vi "PWM Set Phase.vi"(8 "error in (no error)":errorcluster, 9 "pPhase":u16, 10 "ChannelMask":u8, 11 "DevHandle":i32) -> (0 "error out":errorcluster, 1 "pPhase out":u16, 3 "function return":i32)   [LabVIEW 2010, in "usb2pwm.lvlib"]
doc: "int WINAPI PWM_SetPhase(int DevHandle,unsigned char ChannelMask,unsigned short *pPhase);"
uses:
  usb2pwm.lvlib
  libs/msvc_x86/USB2XXX.dll
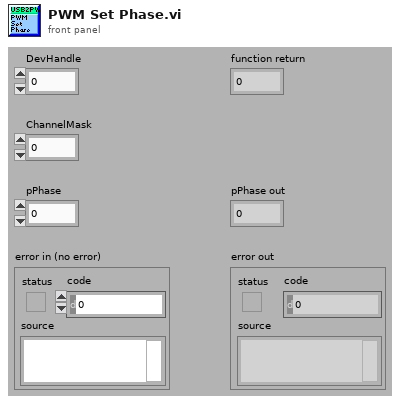
[diagram p1: front panel]
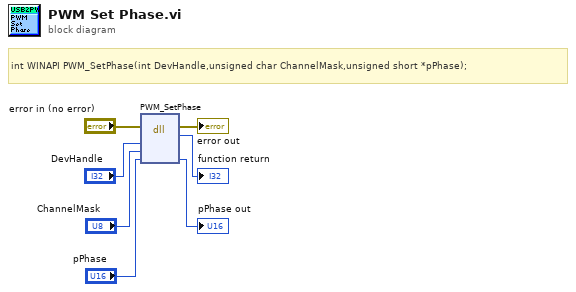
[diagram p0: block diagram]
diagram:
  # "int WINAPI PWM_SetPhase(int DevHandle,unsigned char ChannelMask,unsigned short *pPhase);"
  n1 = dll-call lib="E:/OtherWork/STM32/USB2XXX_Example/sdk/libs/msvc_x86/USB2XXX.*" fn="PWM_SetPhase"(error in="error in (no error)", "DevHandle"="DevHandle", "ChannelMask"="ChannelMask", "pPhase"="pPhase") -> (error out=→"error out":errorcluster, →"function return":i32, "pPhase"=→"pPhase out":u16)  [unwired: 4 in, 1 out]
